vi ".vi"(0 "Reset Counter":bool, 2 "Integral in":dbl format="%#_13g", 5 "Fi":dbl, 7 "Ki":dbl, 9 "Kp":dbl, 11 "Kd":dbl, 12 "PWM freq [Hz] in":dbl) -> (1 "Counter Direction":enum16{"Counting Up", "Counting Down"}(ring), 3 "Counter Value":i32, 4 "Integral out":dbl, 6 "fi":dbl, 10 "dx/dt":dbl, 14 "pwm":dbl, 15 "error out":errorcluster)   [LabVIEW 2019]
uses:
  <vilib>/myRIO/Instrument Drivers/Onboard IO/DIO/typedefs/DIO Reference.ctl
  <vilib>/myRIO/Common/Instrument Driver Framework/Utilities/typedefs/myRIO Generic Hardware Reference.ctl
  <vilib>/myRIO/Common/Instrument Driver Framework/Utilities/typedefs/Hardware Version Enum.ctl
  <vilib>/myRIO/Common/Instrument Driver Framework/Utilities/typedefs/myRIO v1.0 Reference.ctl
  <vilib>/myRIO/Common/Instrument Driver Framework/Utilities/typedefs/Generic FPGA Reference.ctl
  <vilib>/myRIO/Common/Instrument Driver Framework/myRIO v1.0/DIO/typedefs/DIO Channels List.ctl
  <vilib>/myRIO/Common/Instrument Driver Framework/myRIO v1.0/DIO/typedefs/DIO Channels Enum.ctl
  <vilib>/userDefined/High Color/nirio_resource_hc.ctl
  <vilib>/myRIO/Instrument Drivers/Onboard IO/PWM/typedefs/PWM Reference.ctl
  <vilib>/myRIO/Common/Instrument Driver Framework/myRIO v1.0/PWM/typedefs/PWM Channels Enum.ctl
  <vilib>/myRIO/Instrument Drivers/Onboard IO/PWM/typedefs/PWM Configuration.ctl
  <vilib>/myRIO/Common/Instrument Driver Framework/myRIO v1.0/Encoder/typedefs/Encoder Signal Mode.ctl
  <vilib>/myRIO/Instrument Drivers/Onboard IO/Encoder/typedefs/Encoder Reference.ctl
  <vilib>/myRIO/Common/Instrument Driver Framework/myRIO v1.0/Encoder/typedefs/Encoder Channels Enum.ctl
  <vilib>/myRIO/Common/Instrument Driver Framework/myRIO v1.0/Encoder/typedefs/Encoder Configuration v1.0.ctl
  <vilib>/myRIO/Express VI/Onboard IO/DO/DO Express VI.xnode
  <vilib>/myRIO/Instrument Drivers/Onboard IO/DIO/vis/myRIO DIO Open.xnode
  <vilib>/myRIO/Express VI/Onboard IO/PWM/PWM Express VI.xnode
  <vilib>/myRIO/Instrument Drivers/Onboard IO/PWM/vis/myRIO PWM Open.xnode
  <vilib>/myRIO/Express VI/Onboard IO/Encoder/Encoder Express VI.xnode
  <vilib>/myRIO/Common/Instrument Driver Framework/myRIO v1.0/Encoder/typedefs/Encoder Count Direction Enum.ctl
  <vilib>/myRIO/Instrument Drivers/Onboard IO/Encoder/vis/myRIO Encoder Open.xnode
  <vilib>/ptbypt/NI_PtbyPt.lvlib
  <vilib>/myRIO/Instrument Drivers/Onboard IO/Encoder/Encoder.lvlib
  <vilib>/myRIO/Instrument Drivers/Onboard IO/DIO/DIO.lvlib
  <vilib>/myRIO/Instrument Drivers/Onboard IO/PWM/PWM.lvlib
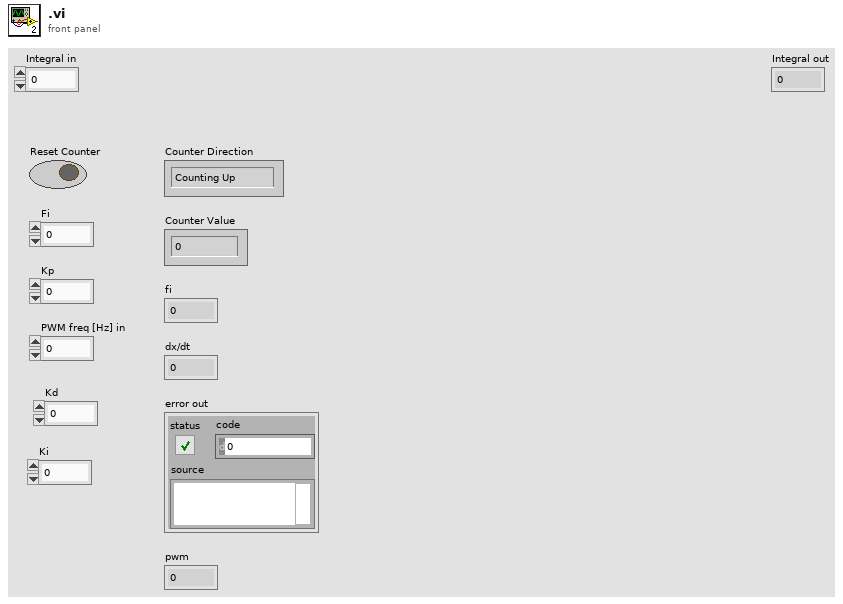
[diagram p1: front panel]
types:
  T1 = typedef "Encoder Count Direction Enum.ctl" = enum16{"Counting Up", "Counting Down"}
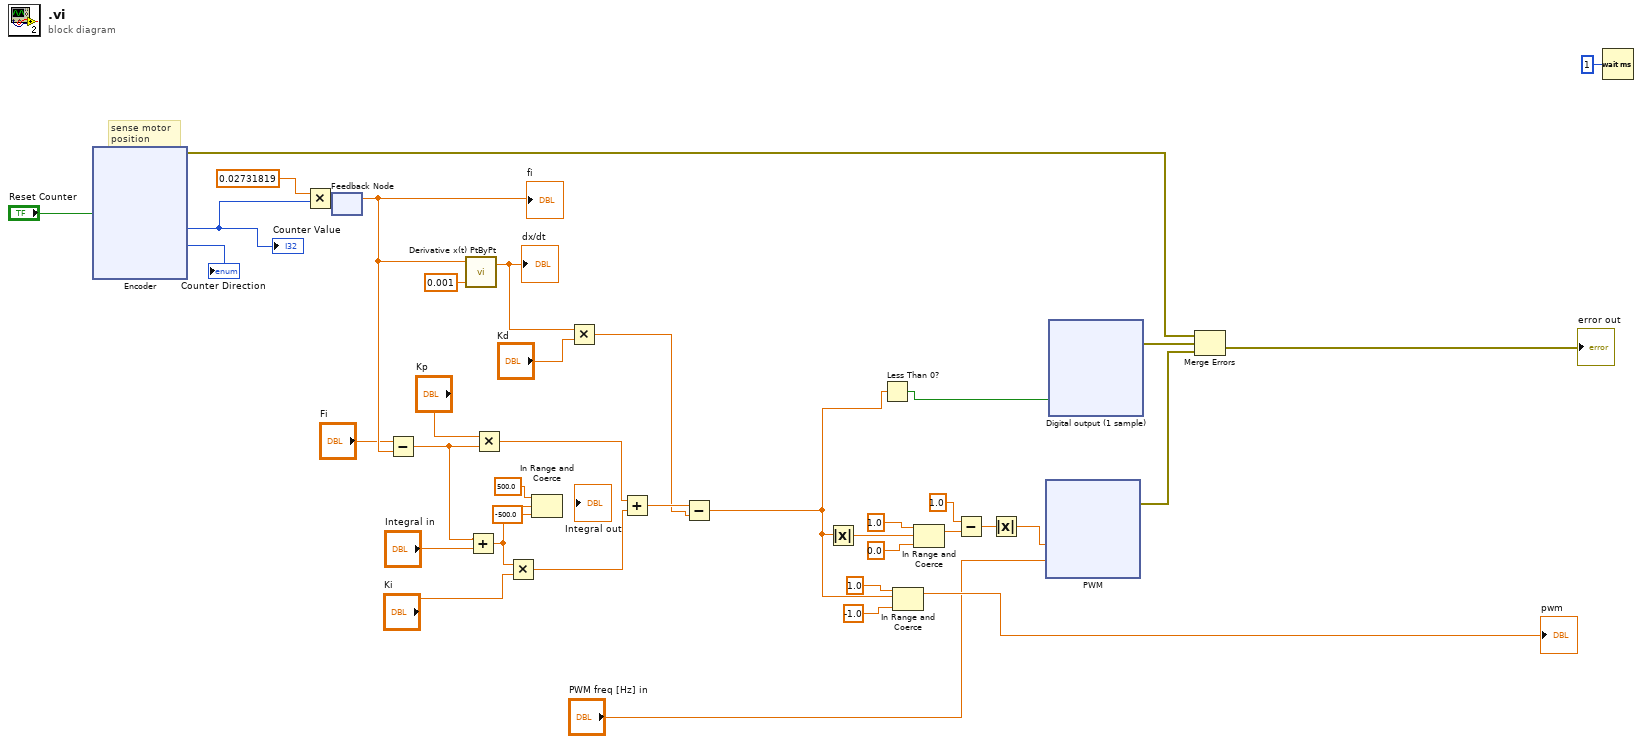
[diagram p0: block diagram]
diagram:
  # "sense motor \nposition"
  n1 = xnode "Encoder"("Reset Counter"="Reset Counter") -> ("Counter Value"=w26:i32, "Counter Direction"=→"Counter Direction":T1, "error out"=w18:errorcluster)  [unwired: 1 in, 1 out]
  "Counter Value" <- w26
  n2 = Multiply(x=0.02731819, y=w26) -> (x*y=w25:dbl)
  n3 = feedback #1() -> (w6:dbl)  [unwired: 1 in]
  "fi" <- w6
  n4 = feedback-in #1(w25) -> ()
  n5 = Subtract(x="Fi", y=w6) -> (x-y=w15:dbl)
  n6 = call <vilib>:"Derivative x(t) PtByPt.vi"("dt"=0.001, "x"=w6) -> ("dx/dt"=w13:dbl)  [unwired: 2 in, 1 out]
  "dx/dt" <- w13
  n7 = Add(x=w15, y="Integral in") -> (x+y=w4:dbl)
  n8 = Multiply(x="Kp", y=w15) -> (x*y=w10:dbl)
  n9 = Multiply(x=w4, y="Ki") -> (x*y=w11:dbl)
  n10 = In Range and Coerce(upper limit=500.0, x=w4, lower limit=-500.0) -> ()  [unwired: 2 out]
  n11 = Multiply(x=w13, y="Kd") -> (x*y=w8:dbl)
  n12 = Add(x=w10, y=w11) -> (x+y=w9:dbl)
  n13 = Subtract(x=w9, y=w8) -> (x-y=w7:dbl)
  n14 = Absolute Value(x=w7) -> (abs(x)=w36:dbl)
  n15 = Less Than 0?(x=w7) -> (x < 0?=w1:bool)
  n16 = In Range and Coerce(upper limit=1.0, x=w7, lower limit=-1.0) -> (coerced(x)=→"pwm":dbl)  [unwired: 1 out]
  n17 = In Range and Coerce(upper limit=1.0, x=w36, lower limit=0.0) -> (coerced(x)=w35:dbl)  [unwired: 1 out]
  n18 = Subtract(x=1.0, y=w35) -> (x-y=w33:dbl)
  n19 = Absolute Value(x=w33) -> (abs(x)=w34:dbl)
  n20 = xnode "PWM"("Duty Cycle"=w34, "Frequency [Hz]"="PWM freq [Hz] in") -> ("error out"=w28:errorcluster)  [unwired: 1 in]
  n21 = xnode "Digital output (1 sample)"("DIR0 (A/DIO10 (Pin 31))"=w1) -> ("error out"=w21:errorcluster)  [unwired: 1 in]
  n22 = Merge Errors(w18, w21, w28) -> (→"error out":errorcluster)
  n23 = Wait (ms)(milliseconds to wait=u32 1) -> ()  [unwired: 1 out]
